vi "apply data indices.vi"(8 "error in":errorcluster, 10 "index type defs":T1, 11 "fixed channel runtime in":refnum<class "fixed channel runtime.lvclass">) -> (0 "error out":errorcluster, 3 "fixed channel runtime out":refnum<class "fixed channel runtime.lvclass">)   [LabVIEW 2013, in "fixed channel runtime.lvclass"]
uses:
  fixed channel runtime.lvclass
  configuration/index type definitions.ctl
  configuration/fixed channel configuration.lvclass
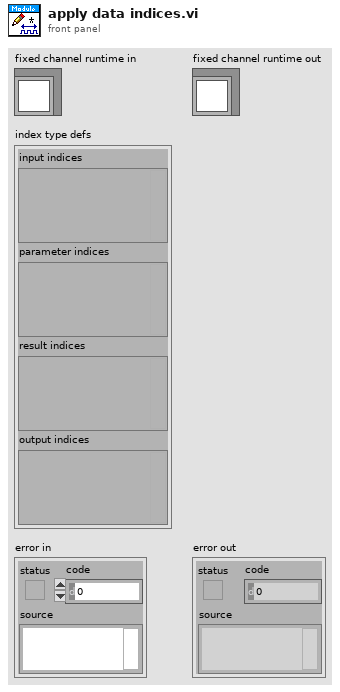
[diagram p1: front panel]
types:
  T1 = typedef "fixed channel configuration.lvclass/index type definitions.ctl" = cluster{"input indices":variant, "parameter indices":variant, "result indices":variant, "output indices":variant}
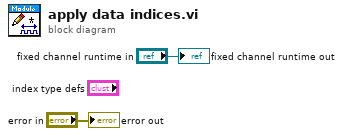
[diagram p0: block diagram]
diagram:
  "error out" <- "error in"
  "fixed channel runtime out" <- "fixed channel runtime in"
